vi "CTRE_Phoenix_MotorControl_ConfigAllSettingsEnhanced.vi"(6 "timeoutMs":i32=50, 7 "Force Write":bool, 8 "error in (no error)":errorcluster, 10 "Enhanced Motor Controller Configurables":T1={"Base Configurables"={"openLoopRamp"=0.0, "closedLoopRamp"=0.0, "peakOutputForward"=1.0, "peakOutputReverse"=-1.0, "nominalOutputForward"=0.0, "nominalOutputReverse"=0.0, "neutralDeadband"=0.04, "voltageCompSaturation"=0.0, "voltageMeasurementFilter"=32, "velocityMeasurementPeriod"=100, "velocityMeasurementWindow"=64, "forwardSoftLimitThreshold"=0, "reverseSoftLimitThreshold"=0, "forwardSoftLimitEnable"=FALSE, "reverseSoftLimitEnable"=FALSE, "slot0"={"P"=0.0, "I"=0.0, "D"=0.0, "F"=0.0, "integralZone"=0.0, "allowableClosedLoopError"=0, "maxIntegralAccumulator"=0.0, "closedLoopPeakOutput"=1.0, "closedLoopPeriod"=1}, "slot1"={"P"=0.0, "I"=0.0, "D"=0.0, "F"=0.0, "integralZone"=0.0, "allowableClosedLoopError"=0, "maxIntegralAccumulator"=0.0, "closedLoopPeakOutput"=1.0, "closedLoopPeriod"=1}, "slot2"={"P"=0.0, "I"=0.0, "D"=0.0, "F"=0.0, "integralZone"=0.0, "allowableClosedLoopError"=0, "maxIntegralAccumulator"=0.0, "closedLoopPeakOutput"=1.0, "closedLoopPeriod"=1}, "slot3"={"P"=0.0, "I"=0.0, "D"=0.0, "F"=0.0, "integralZone"=0.0, "allowableClosedLoopError"=0, "maxIntegralAccumulator"=0.0, "closedLoopPeakOutput"=1.0, "closedLoopPeriod"=1}, "auxPIDPolarity"=FALSE, "remoteFilter0"={"remoteSensorDeviceID"=0, "remoteSensorSource"=enum."Off"}, "remoteFilter1"={"remoteSensorDeviceID"=0, "remoteSensorSource"=enum."Off"}, "motionCruiseVelocity"=0, "motionAcceleration"=0, "motionProfileTrajectoryPeriod"=0, "feedbackNotContinuous"=FALSE, "remoteSensorClosedLoopDisableNeutralOnLOS"=FALSE, "clearPositionOnLimitF"=FALSE, "clearPositionOnLimitR"=FALSE, "clearPositionOnQuadIdx"=FALSE, "limitSwitchDisableNeutralOnLOS"=FALSE, "softLimitDisableNeutralOnLOS"=FALSE, "pulseWidthPeriod_EdgesPerRot"=1, "pulseWidthPeriod_FilterWindowSz"=1, "customParam"={"customParam0"=0, "customParam1"=0}}, "primaryPID"={"selectedFeedbackCoefficient"=1.0, "selectedFeedbackSensor"=0}, "auxiliaryPID"={"selectedFeedbackCoefficient"=1.0, "selectedFeedbackSensor"=0}, "sum0Term"=0, "sum1Term"=0, "diff0Term"=0, "diff1Term"=0, "forwardLimitSwitchNormal"=enum."Normally Open", "reverseLimitSwitchNormal"=enum."Normally Open", "forwardLimitSwitchDeviceID"=0, "reverseLimitSwitchDeviceID"=0, "forwardLimitSwitchSource"=enum."Feedback Connector", "reverseLimitSwitchSource"=enum."Feedback Connector", "peakCurrentLimit"=1, "peakCurrentDuration"=1, "continuousCurrentLimit"=1} {"diff1Term" items=["QuadEncoder"=0, "Analog"=2, "Tachometer"=4, "Pulse Width Encoded Position"=8, "Remote Source 0"=11, "Remote Source 1"=12, "Software Emulated"=15]; "diff0Term" items=["QuadEncoder"=0, "Analog"=2, "Tachometer"=4, "Pulse Width Encoded Position"=8, "Remote Source 0"=11, "Remote Source 1"=12, "Software Emulated"=15]; "sum1Term" items=["QuadEncoder"=0, "Analog"=2, "Tachometer"=4, "Pulse Width Encoded Position"=8, "Remote Source 0"=11, "Remote Source 1"=12, "Software Emulated"=15]; "sum0Term" items=["QuadEncoder"=0, "Analog"=2, "Tachometer"=4, "Pulse Width Encoded Position"=8, "Remote Source 0"=11, "Remote Source 1"=12, "Software Emulated"=15]; "auxiliaryPID"."selectedFeedbackSensor" items=["QuadEncoder"=0, "Analog"=2, "Tachometer"=4, "Pulse Width Encoded Position"=8, "Sensor Sum (S0 + S1)"=9, "Sensor Difference (D0 - D1)"=10, "Remote Source 0"=11, "Remote Source 1"=12, "Software Emulated"=15]; "primaryPID"."selectedFeedbackSensor" items=["QuadEncoder"=0, "Analog"=2, "Tachometer"=4, "Pulse Width Encoded Position"=8, "Sensor Sum (S0 + S1)"=9, "Sensor Difference (D0 - D1)"=10, "Remote Source 0"=11, "Remote Source 1"=12, "Software Emulated"=15]; "Base Configurables"."velocityMeasurementPeriod" items=["Period_1ms"=1, "Period_2ms"=2, "Period_5ms"=5, "Period_10ms"=10, "Period_20ms"=20, "Period_25ms"=25, "Period_50ms"=50, "Period_100ms"=100]}, 11 "PhoenixMotorControlDevRef":T12={"DeviceStatus"={"status"=FALSE, "code"=0, "source"=""}, "Type"=enum."PWM", "PWM"={"PWM Channel"=enum."PWM 1", "DeadBand"={"Name"="", "maxPositivePwm"=0, "minPositivePwm"=0, "centerPwm"=0, "maxNegativePwm"=0, "minNegativePwm"=0, "angularRange"=0}}, "CAN"={"Device Number"=0, "SetOutput VI Ref"=variant(enum8{"Percent VBus", "Current", "Speed", "Position", "Voltage"} enum."Percent VBus"), "GetOutput VI Ref"=variant(refnum<k1> refnum), "Enable VI Ref"=variant(dbl 12.0), "Disable VI Ref"=variant(enum8{"Percent VBus", "Speed", "Position", "Slave", "Unchanged / Invalid", "Voltage Compensation", "Current", "Motion Profile"} enum."Percent VBus"), "Data"=variant}, "Invert"=FALSE, "DIO PWM"={"PWM \"Enable\" Channel"=enum."Invalid", "DIOChannel"=enum."Invalid", "PWM Rate"=0.0}}) -> (0 "error out":errorcluster, 3 "PhoenixMotorControlDevRef":T12={"DeviceStatus"={"status"=FALSE, "code"=0, "source"=""}, "Type"=enum."PWM", "PWM"={"PWM Channel"=enum."PWM 1", "DeadBand"={"Name"="", "maxPositivePwm"=0, "minPositivePwm"=0, "centerPwm"=0, "maxNegativePwm"=0, "minNegativePwm"=0, "angularRange"=0}}, "CAN"={"Device Number"=0, "SetOutput VI Ref"=variant(enum8{"Percent VBus", "Current", "Speed", "Position", "Voltage"} enum."Percent VBus"), "GetOutput VI Ref"=variant(refnum<k1> refnum), "Enable VI Ref"=variant(dbl 12.0), "Disable VI Ref"=variant(enum8{"Percent VBus", "Speed", "Position", "Slave", "Unchanged / Invalid", "Voltage Compensation", "Current", "Motion Profile"} enum."Percent VBus"), "Data"=variant}, "Invert"=FALSE, "DIO PWM"={"PWM \"Enable\" Channel"=enum."Invalid", "DIOChannel"=enum."Invalid", "PWM Rate"=0.0}})   [LabVIEW 2017]
doc: "Configures all slot persistant settings\n\n<b> Enhanced Motor Controller Configurables </b> Cluster of all settinsg to be configured"
uses:
  <vilib>/Rock Robotics/WPI/MotorControl/WPI_MotorControlDeviceRef.ctl
  <vilib>/Rock Robotics/WPI/MotorControl/WPI_MotorControlType.ctl
  <vilib>/Rock Robotics/SystemInterfaces/DIO/FPGA_DIOPWMChannel.ctl
  <vilib>/Rock Robotics/WPI/PWM/WPI_PWMDeadband.ctl
  <vilib>/Rock Robotics/SystemInterfaces/DIO/FPGA_DIOChannel.ctl
  <vilib>/Rock Robotics/WPI/ThirdParty/Phoenix-LabVIEW/Motor Controller/Controls/CTRE_Phoenix_MotorControl_EnhancedMotorControllerConfigurables.ctl
  <vilib>/Rock Robotics/WPI/ThirdParty/Phoenix-LabVIEW/Motor Controller/Controls/CTRE_Phoenix_MotorControl_BaseConfigurables.ctl
  <vilib>/Rock Robotics/WPI/ThirdParty/Phoenix-LabVIEW/Motor Controller/Controls/CTRE_Phoenix_MotorControl_VelocityMeasurementPeriod.ctl
  <vilib>/Rock Robotics/WPI/ThirdParty/Phoenix-LabVIEW/Motor Controller/Controls/CTRE_Phoenix_MotorControl_SlotStructure.ctl
  <vilib>/Rock Robotics/WPI/ThirdParty/Phoenix-LabVIEW/Motor Controller/Controls/CTRE_Phoenix_MotorControl_FilterStruct.ctl
  <vilib>/Rock Robotics/WPI/ThirdParty/Phoenix-LabVIEW/Motor Controller/Controls/CTRE_Phoenix_MotorControl_RemoteSourceType.ctl
  <vilib>/Rock Robotics/WPI/ThirdParty/Phoenix-LabVIEW/Controls/CTRE_Phoenix_CustomParamConfiguration.ctl
  <vilib>/Rock Robotics/WPI/ThirdParty/Phoenix-LabVIEW/Motor Controller/Controls/CTRE_Phoenix_MotorControl_FeedbackDevice.ctl
  <vilib>/Rock Robotics/WPI/ThirdParty/Phoenix-LabVIEW/Motor Controller/Controls/CTRE_Phoenix_MotorControl_SensorTermFeedbackDevice_Enhanced.ctl
  <vilib>/Rock Robotics/WPI/ThirdParty/Phoenix-LabVIEW/Motor Controller/Controls/CTRE_Phoenix_MotorControl_LimitSwitchNormal.ctl
  <vilib>/Rock Robotics/WPI/ThirdParty/Phoenix-LabVIEW/Motor Controller/Controls/CTRE_Phoenix_MotorControl_LimitSwitchSource_Local.ctl
panel:
  # "Sum and Diff terms are ways to select more than one sensor as a feedback device. \n Sum 0 is the first feedback device to be used for the Sum term.\n Sum 1 is the feedback device to be added to Sum 0 for the Sum term.\n Diff 0 and Diff 1 work in a similar manner."
  # "These are only applicable\nif using a remote limit switch.\n\nLocal limit switches/no limit\nswitches do not use this."
  # "Current is below Continuous threshold AND\n\n(Requested output is weaker** than applied motor\noutput OR is in the opposite direction).\n/\nMotor output is set to requested output."
  # "Current is above Peak* Threshold for Peak Duration.\n/\nReduce motor output (towards neutral)."
  # "Current is below Continuous threshold.\n/\nRamp motor output towards requested output."
  # "Current is above Continuous threshold.\n/\nReduce motor output (towards neutral)."
  # "Current Limiting is NOT enabled\nby default.\nCall this VI to enable."
  # "*If the configured Peak Threshold is less than the Continuous Threshold, the applied Peak Threshold is set equal to the Configured Continuous Threshold in firmware.\n** Both requested output and applied motor output are in the same direction, and requested output is closer to neutral."
  # "False: Primary Output = PID[0] + PID[1]  ---  Auxiliary Output = PID[0] - PID[1]\nTrue:  Primary Output = PID[0] - PID[1] --- Auxiliary Output = PID[0] + PID[1]"
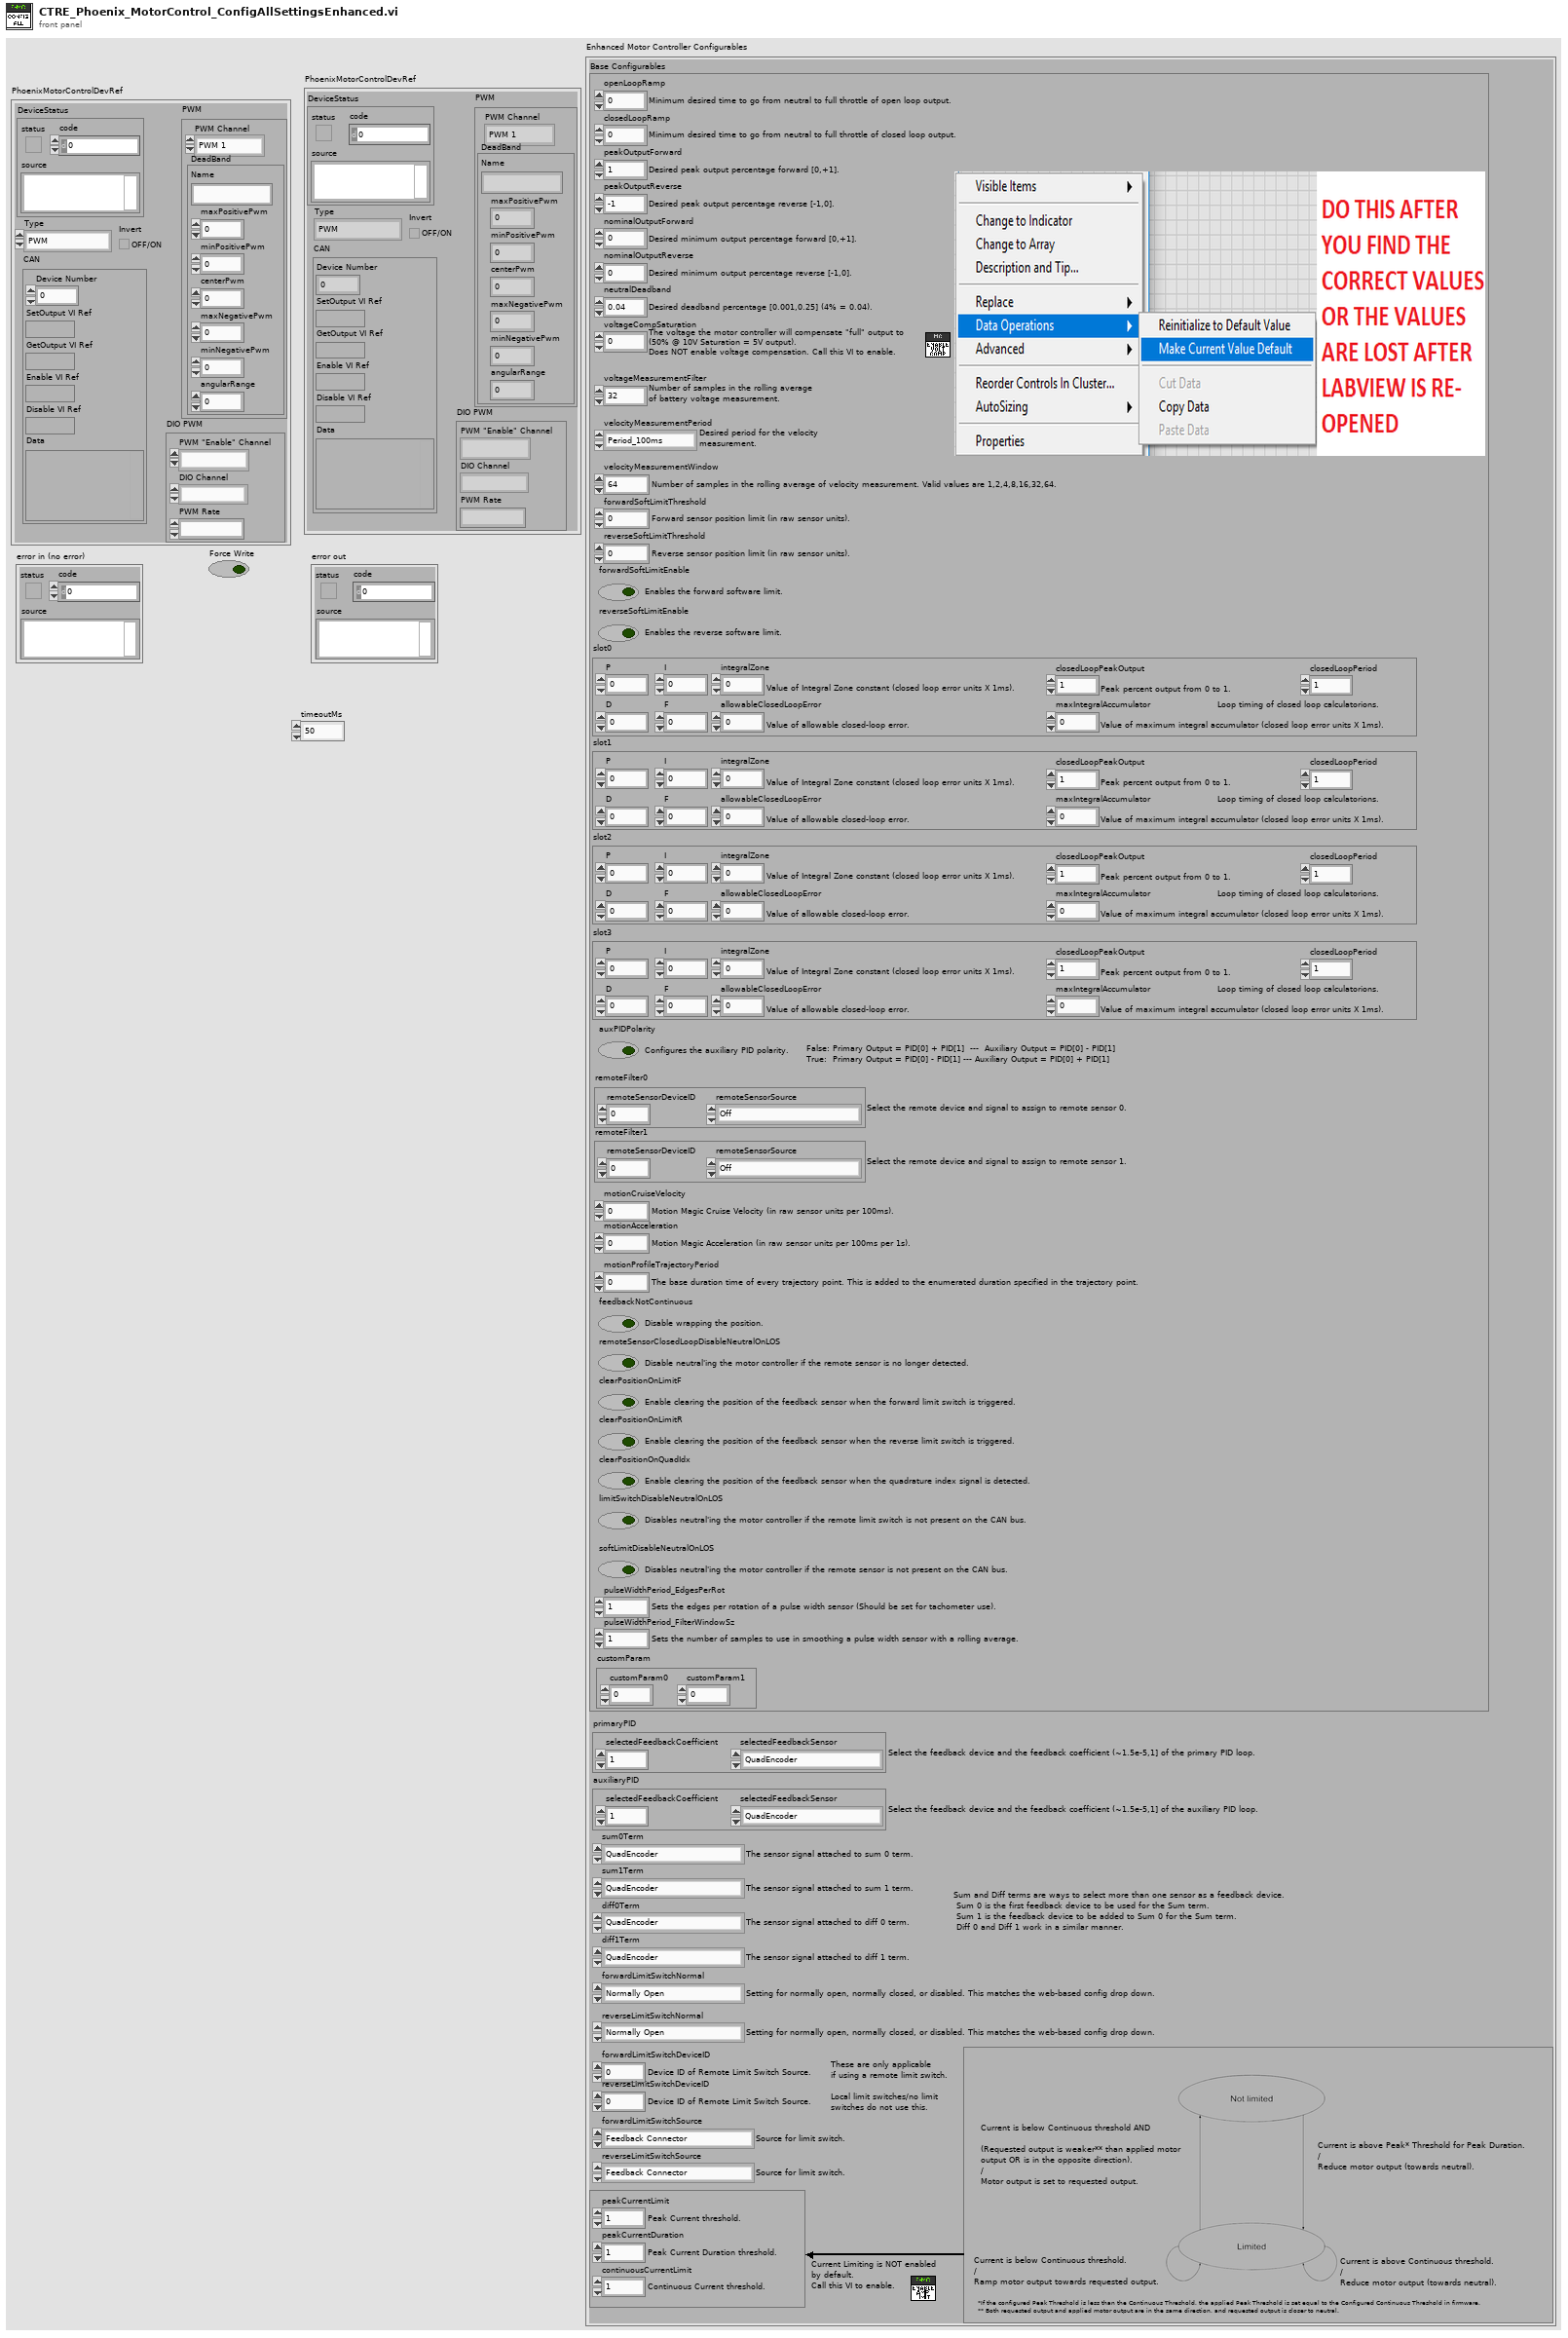
[diagram p1: front panel]
types:
  T1 = typedef "CTRE_Phoenix_MotorControl_EnhancedMotorControllerConfigurables.ctl" = cluster{"Base Configurables":T2, "primaryPID":cluster{"selectedFeedbackCoefficient":dbl, "selectedFeedbackSensor":T8}, "auxiliaryPID":cluster{"selectedFeedbackCoefficient":dbl, "selectedFeedbackSensor":T8}, "sum0Term":T9, "sum1Term":T9, "diff0Term":T9, "diff1Term":T9, "forwardLimitSwitchNormal":T10, "reverseLimitSwitchNormal":T10, "forwardLimitSwitchDeviceID":i32, "reverseLimitSwitchDeviceID":i32, "forwardLimitSwitchSource":T11, "reverseLimitSwitchSource":T11, "peakCurrentLimit":i32, "peakCurrentDuration":i32, "continuousCurrentLimit":i32}
  T2 = typedef "CTRE_Phoenix_MotorControl_BaseConfigurables.ctl" = cluster{"openLoopRamp":dbl, "closedLoopRamp":dbl, "peakOutputForward":dbl, "peakOutputReverse":dbl, "nominalOutputForward":dbl, "nominalOutputReverse":dbl, "neutralDeadband":dbl, "voltageCompSaturation":dbl, "voltageMeasurementFilter":i32, "velocityMeasurementPeriod":T3, "velocityMeasurementWindow":i32, "forwardSoftLimitThreshold":i32, "reverseSoftLimitThreshold":i32, "forwardSoftLimitEnable":bool, "reverseSoftLimitEnable":bool, "slot0":T4, "slot1":T4, "slot2":T4, "slot3":T4, "auxPIDPolarity":bool, "remoteFilter0":T5, "remoteFilter1":T5, "motionCruiseVelocity":i32, "motionAcceleration":i32, "motionProfileTrajectoryPeriod":i32, "feedbackNotContinuous":bool, "remoteSensorClosedLoopDisableNeutralOnLOS":bool, "clearPositionOnLimitF":bool, "clearPositionOnLimitR":bool, "clearPositionOnQuadIdx":bool, "limitSwitchDisableNeutralOnLOS":bool, "softLimitDisableNeutralOnLOS":bool, "pulseWidthPeriod_EdgesPerRot":i32, "pulseWidthPeriod_FilterWindowSz":i32, "customParam":T7}
  T3 = typedef "CTRE_Phoenix_MotorControl_VelocityMeasurementPeriod.ctl" = u16
  T4 = typedef "CTRE_Phoenix_MotorControl_SlotStructure.ctl" = cluster{"P":dbl, "I":dbl, "D":dbl, "F":dbl, "integralZone":dbl, "allowableClosedLoopError":i32, "maxIntegralAccumulator":dbl, "closedLoopPeakOutput":dbl, "closedLoopPeriod":i32}
  T5 = typedef "CTRE_Phoenix_MotorControl_FilterStruct.ctl" = cluster{"remoteSensorDeviceID":u8, "remoteSensorSource":T6}
  T6 = typedef "CTRE_Phoenix_MotorControl_RemoteSourceType.ctl" = enum16{"Off", "Talon SRX Selected Sensor", "Pigeon IMU Yaw", "Pigeon IMU Pitch", "Pigeon IMU Roll", "CANifier Quadrature", "CANifier PWM Input 0", "CANifier PWM Input 1", "CANifier PWM Input 2", "CANifier PWM Input 3", "Gadgeteer Pigeon Yaw", "Gadgeteer Pigeon Pitch", "Gadgeteer Pigeon Roll"}
  T7 = typedef "CTRE_Phoenix_CustomParamConfiguration.ctl" = cluster{"customParam0":i32, "customParam1":i32}
  T8 = typedef "CTRE_Phoenix_MotorControl_FeedbackDevice.ctl" = i8
  T9 = typedef "CTRE_Phoenix_MotorControl_SensorTermFeedbackDevice_Enhanced.ctl" = i8
  T10 = typedef "CTRE_Phoenix_MotorControl_LimitSwitchNormal.ctl" = enum16{"Normally Open", "Normally Closed", "Disabled"}
  T11 = typedef "CTRE_Phoenix_MotorControl_LimitSwitchSource_Local.ctl" = enum16{"Feedback Connector", "Remote Talon SRX", "Remote CANifier", "Deactivated"}
  T12 = typedef "WPI_MotorControlDeviceRef.ctl" = cluster{"DeviceStatus":errorcluster, "Type":T13, "PWM":cluster{"PWM Channel":T14, "DeadBand":T15}, "CAN":cluster{"Device Number":u8, "SetOutput VI Ref":variant, "GetOutput VI Ref":variant, "Enable VI Ref":variant, "Disable VI Ref":variant, "Data":variant}, "Invert":bool, "DIO PWM":cluster{"PWM \"Enable\" Channel":T14, "DIOChannel":T16, "PWM Rate":dbl}}
  T13 = typedef "WPI_MotorControlType.ctl" = enum16{"PWM", "CAN", "DIO PWM"}
  T14 = typedef "FPGA_DIOPWMChannel.ctl" = enum8{"PWM 0", "PWM 1", "PWM 2", "PWM 3", "PWM 4", "PWM 5", "PWM 6", "PWM 7", "PWM 8", "PWM 9", "PWM MXP 0", "PWM MXP 1", "PWM MXP 2", "PWM MXP 3", "PWM MXP 4", "PWM MXP 5", "PWM MXP 6", "PWM MXP 7", "PWM MXP 8", "PWM MXP 9", "Invalid"}
  T15 = typedef "WPI_PWMDeadband.ctl" = cluster{"Name":string, "maxPositivePwm":i32, "minPositivePwm":i32, "centerPwm":i32, "maxNegativePwm":i32, "minNegativePwm":i32, "angularRange":u16}
  T16 = typedef "FPGA_DIOChannel.ctl" = enum8{"DIO 0", "DIO 1", "DIO 2", "DIO 3", "DIO 4", "DIO 5", "DIO 6", "DIO 7", "DIO 8", "DIO 9", "DIO MXP 0", "DIO MXP 1", "DIO MXP 2", "DIO MXP 3", "DIO MXP 4", "DIO MXP 5", "DIO MXP 6", "DIO MXP 7", "DIO MXP 8", "DIO MXP 9", "DIO MXP 10", "DIO MXP 11", "DIO MXP 12", "DIO MXP 13", "DIO MXP 14", "DIO MXP 15", "SPI Port CS1", "SPI Port CS2", "SPI Port CS3", "SPI Port MISO", "SPI Port MOSI", "Invalid"}
  T17 = cluster{"Base Configurables":cluster{"openLoopRamp":bool, "closedLoopRamp":bool, "peakOutputForward":bool, "peakOutputReverse":bool, "nominalOutputForward":bool, "nominalOutputReverse":bool, "neutralDeadband":bool, "voltageCompSaturation":bool, "voltageMeasurementFilter":bool, "velocityMeasurementPeriod":bool, "velocityMeasurementWindow":bool, "forwardSoftLimitThreshold":bool, "reverseSoftLimitThreshold":bool, "forwardSoftLimitEnable":bool, "reverseSoftLimitEnable":bool, "slot0":cluster{"P":bool, "I":bool, "D":bool, "F":bool, "integralZone":bool, "allowableClosedLoopError":bool, "maxIntegralAccumulator":bool, "closedLoopPeakOutput":bool, "closedLoopPeriod":bool}, "slot1":cluster{"P":bool, "I":bool, "D":bool, "F":bool, "integralZone":bool, "allowableClosedLoopError":bool, "maxIntegralAccumulator":bool, "closedLoopPeakOutput":bool, "closedLoopPeriod":bool}, "slot2":cluster{"P":bool, "I":bool, "D":bool, "F":bool, "integralZone":bool, "allowableClosedLoopError":bool, "maxIntegralAccumulator":bool, "closedLoopPeakOutput":bool, "closedLoopPeriod":bool}, "slot3":cluster{"P":bool, "I":bool, "D":bool, "F":bool, "integralZone":bool, "allowableClosedLoopError":bool, "maxIntegralAccumulator":bool, "closedLoopPeakOutput":bool, "closedLoopPeriod":bool}, "auxPIDPolarity":bool, "remoteFilter0":cluster{"remoteSensorDeviceID":bool, "remoteSensorSource":bool}, "remoteFilter1":cluster{"remoteSensorDeviceID":bool, "remoteSensorSource":bool}, "motionCruiseVelocity":bool, "motionAcceleration":bool, "motionProfileTrajectoryPeriod":bool, "feedbackNotContinuous":bool, "remoteSensorClosedLoopDisableNeutralOnLOS":bool, "clearPositionOnLimitF":bool, "clearPositionOnLimitR":bool, "clearPositionOnQuadIdx":bool, "limitSwitchDisableNeutralOnLOS":bool, "softLimitDisableNeutralOnLOS":bool, "pulseWidthPeriod_EdgesPerRot":bool, "pulseWidthPeriod_FilterWindowSz":bool, "customParam":cluster{"customParam0":bool, "customParam1":bool}}, "primaryPID":cluster{"selectedFeedbackCoefficient":bool, "selectedFeedbackSensor":bool}, "auxiliaryPID":cluster{"selectedFeedbackCoefficient":bool, "selectedFeedbackSensor":bool}, "sum0Term":bool, "sum1Term":bool, "diff0Term":bool, "diff1Term":bool, "forwardLimitSwitchNormal":bool, "reverseLimitSwitchNormal":bool, "forwardLimitSwitchDeviceID":bool, "reverseLimitSwitchDeviceID":bool, "forwardLimitSwitchSource":bool, "reverseLimitSwitchSource":bool, "peakCurrentLimit":bool, "peakCurrentDuration":bool, "continuousCurrentLimit":bool}
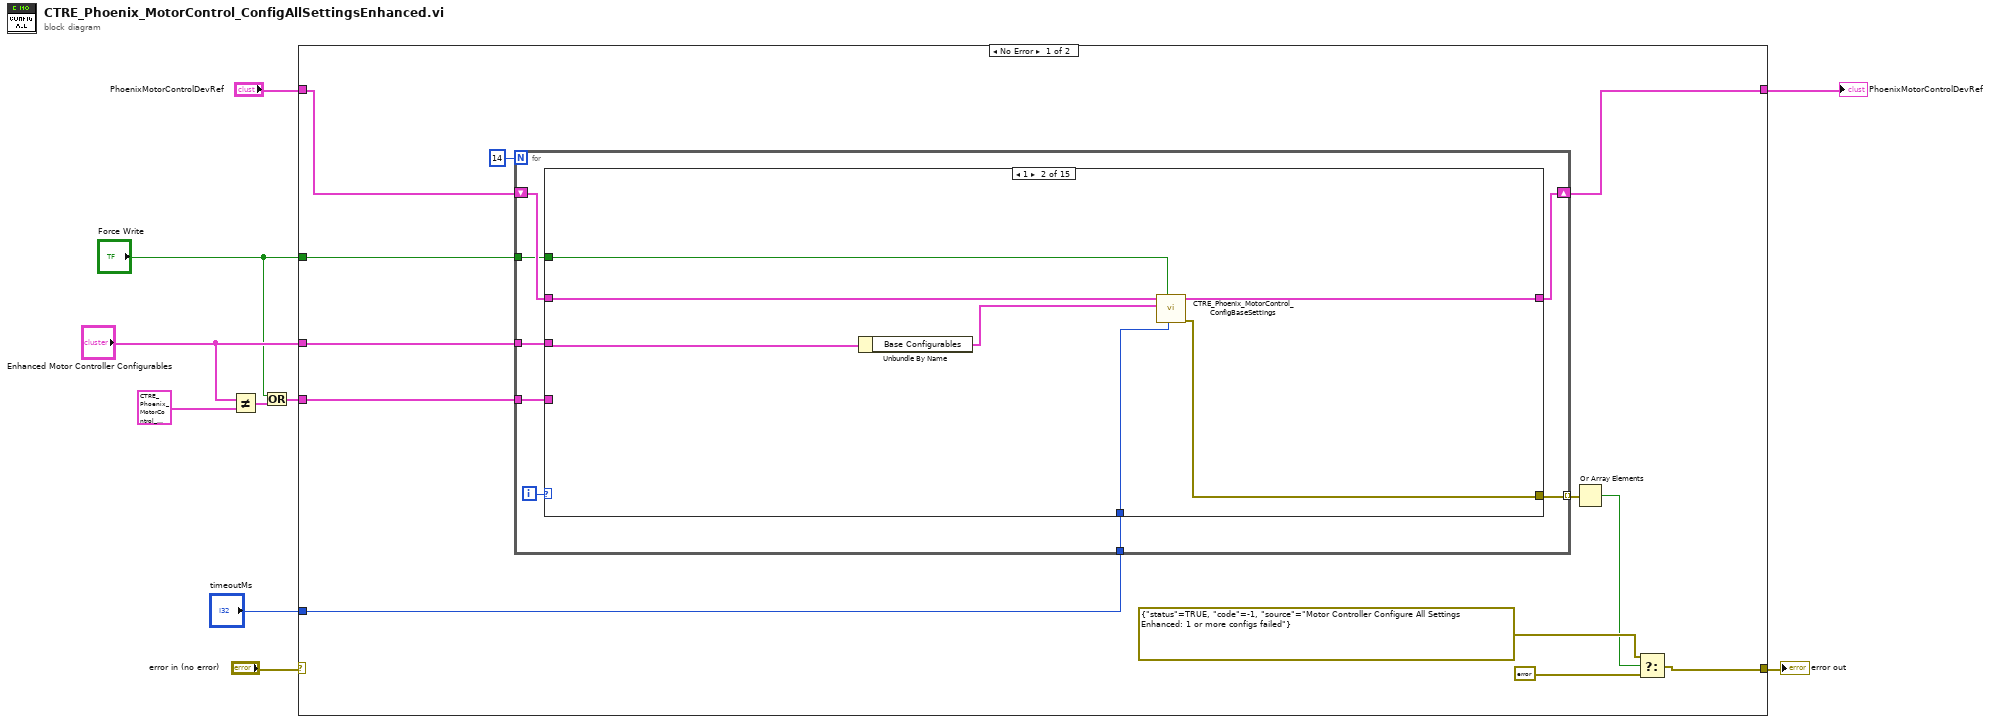
[diagram p0: block diagram]
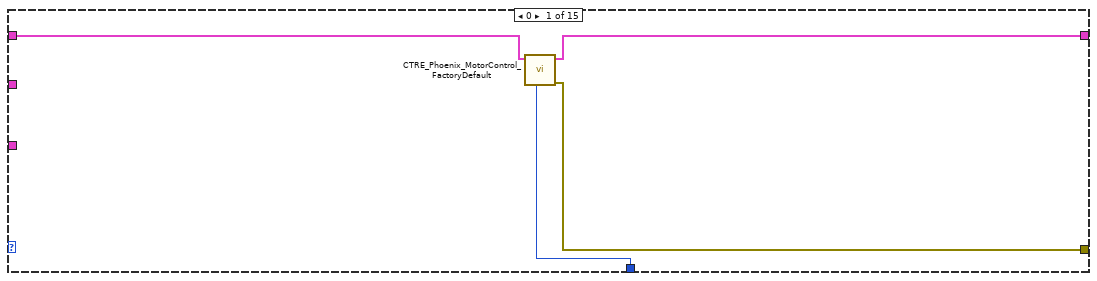
[diagram p2: hidden frame]
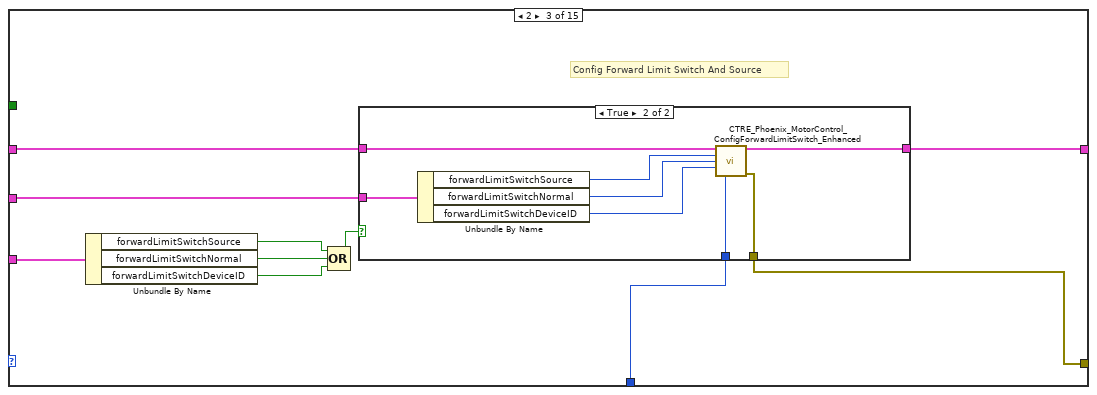
[diagram p3: hidden frame]
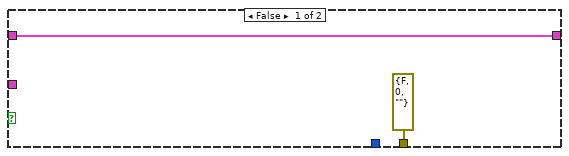
[diagram p4: hidden frame]
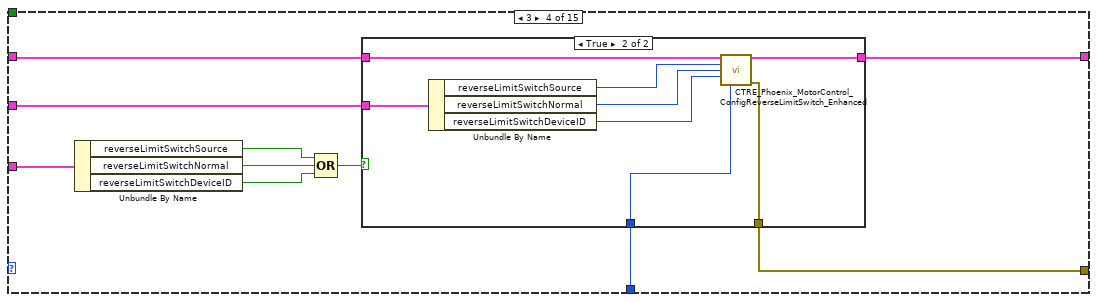
[diagram p5: hidden frame]
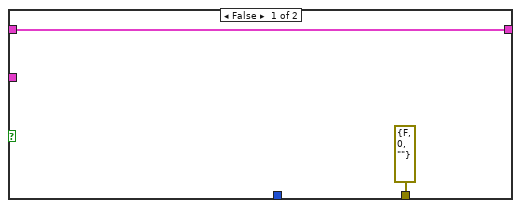
[diagram p6: hidden frame]
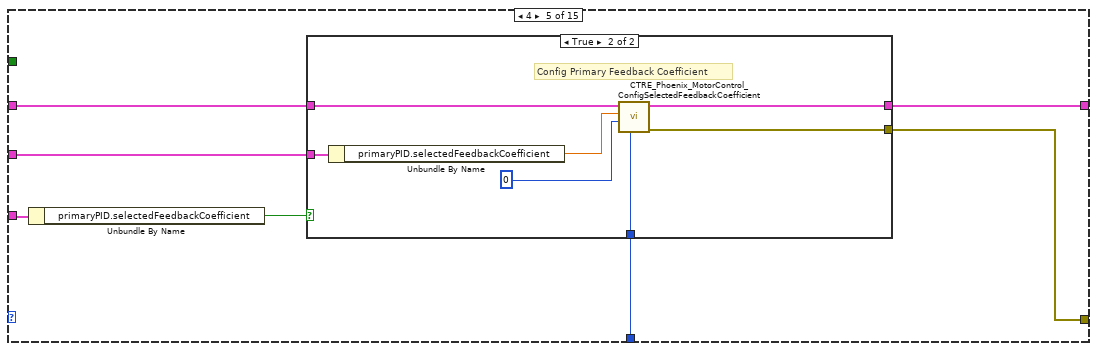
[diagram p7: hidden frame]
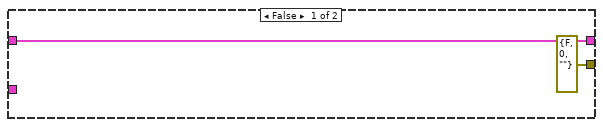
[diagram p8: hidden frame]
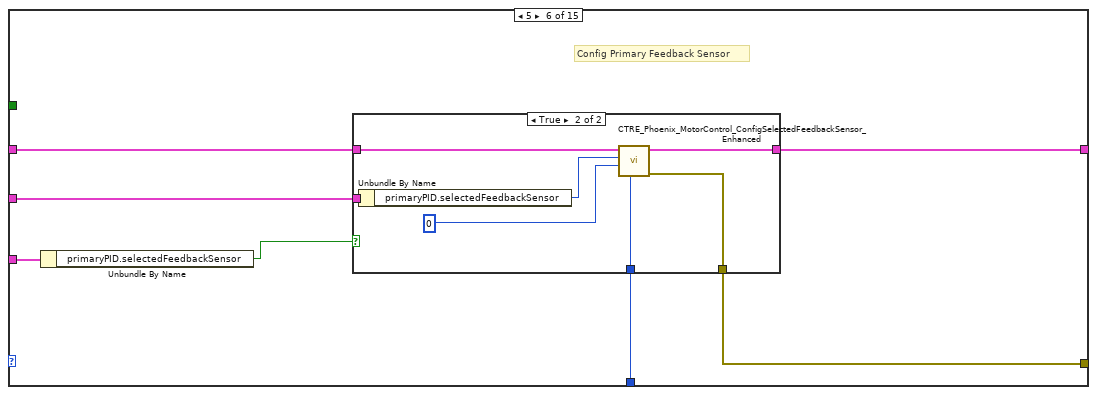
[diagram p9: hidden frame]
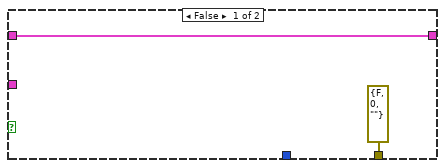
[diagram p10: hidden frame]
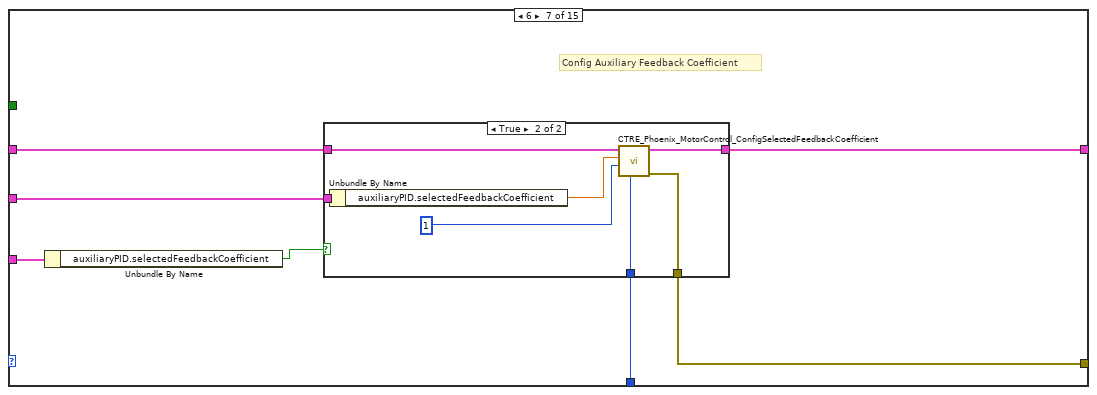
[diagram p11: hidden frame]
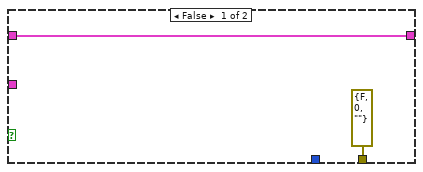
[diagram p12: hidden frame]
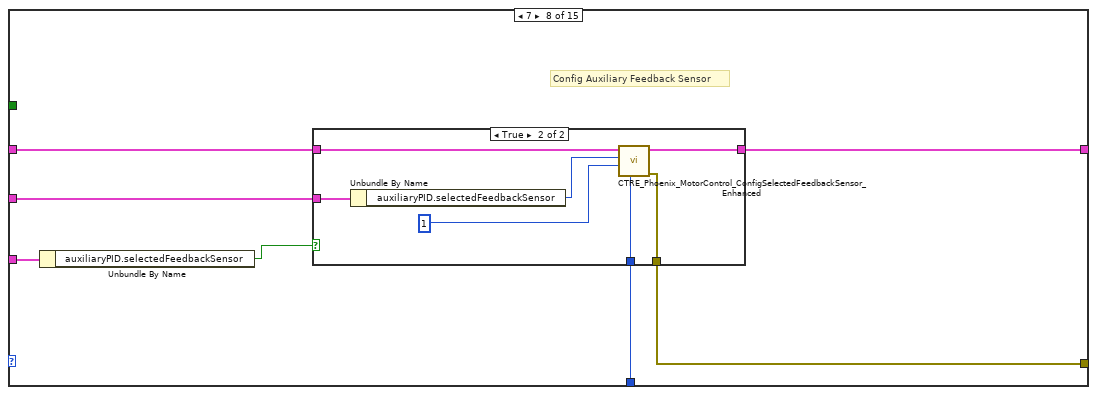
[diagram p13: hidden frame]
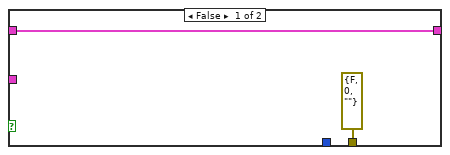
[diagram p14: hidden frame]
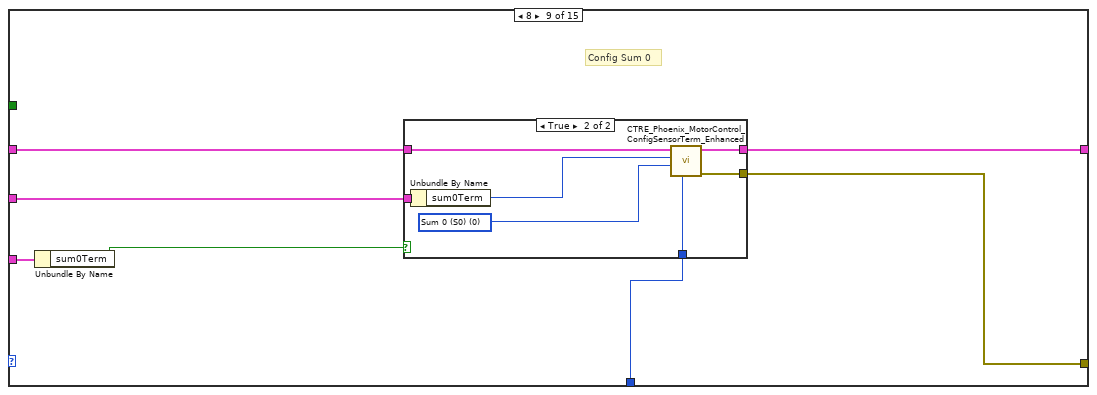
[diagram p15: hidden frame]
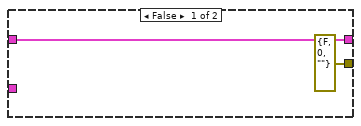
[diagram p16: hidden frame]
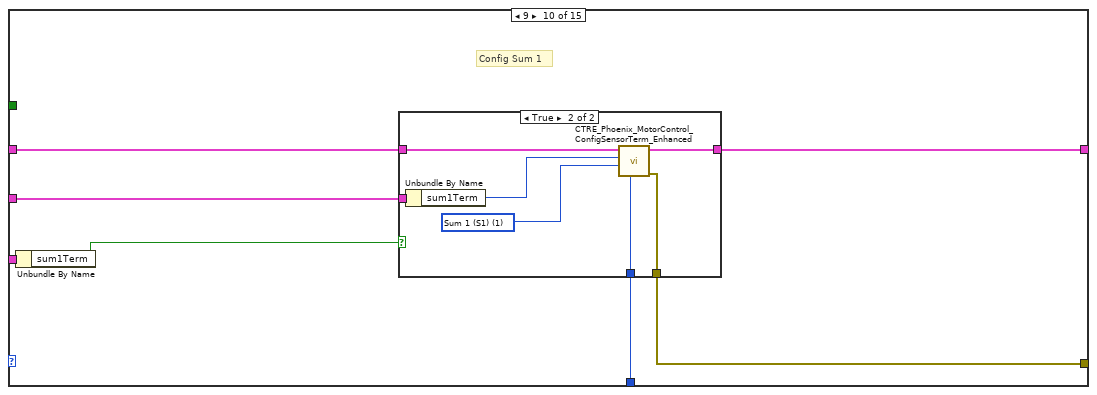
[diagram p17: hidden frame]
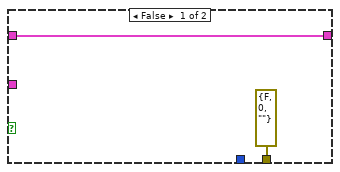
[diagram p18: hidden frame]
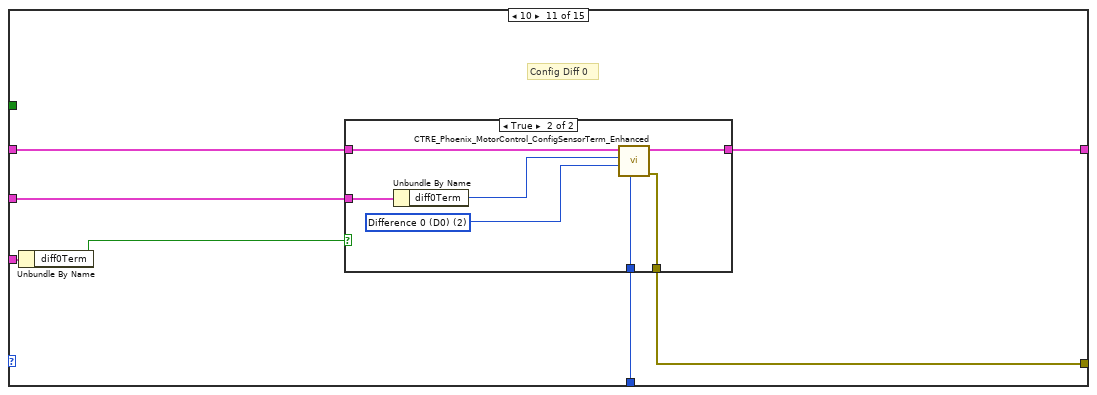
[diagram p19: hidden frame]
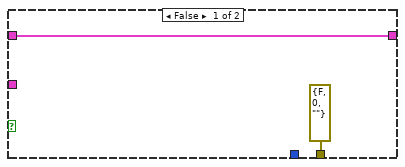
[diagram p20: hidden frame]
diagram:
  n1 = Not Equal?(x="Enhanced Motor Controller Configurables", y=T1 {"Base Configurables"={"openLoopRamp"=0.0, "closedLoopRamp"=0.0, "peakOutputForward"=1.0, "peakOutputReverse"=-1.0, "nominalOutputForward"=0.0, "nominalOutputReverse"=0.0, "neutralDeadband"=0.04, "voltageCompSaturation"=0.0, "voltageMeasurementFilter"=32, "velocityMeasurementPeriod"=100, "velocityMeasurementWindow"=64, "forwardSoftLimitThreshold"=0, "reverseSoftLimitThreshold"=0, "forwardSoftLimitEnable"=FALSE, "reverseSoftLimitEnable"=FALSE, "slot0"={"P"=0.0, "I"=0.0, "D"=0.0, "F"=0.0, "integralZone"=0.0, "allowableClosedLoopError"=0, "maxIntegralAccumulator"=0.0, "closedLoopPeakOutput"=1.0, "closedLoopPeriod"=1}, "slot1"={"P"=0.0, "I"=0.0, "D"=0.0, "F"=0.0, "integralZone"=0.0, "allowableClosedLoopError"=0, "maxIntegralAccumulator"=0.0, "closedLoopPeakOutput"=1.0, "closedLoopPeriod"=1}, "slot2"={"P"=0.0, "I"=0.0, "D"=0.0, "F"=0.0, "integralZone"=0.0, "allowableClosedLoopError"=0, "maxIntegralAccumulator"=0.0, "closedLoopPeakOutput"=1.0, "closedLoopPeriod"=1}, "slot3"={"P"=0.0, "I"=0.0, "D"=0.0, "F"=0.0, "integralZone"=0.0, "allowableClosedLoopError"=0, "maxIntegralAccumulator"=0.0, "closedLoopPeakOutput"=1.0, "closedLoopPeriod"=1}, "auxPIDPolarity"=FALSE, "remoteFilter0"={"remoteSensorDeviceID"=0, "remoteSensorSource"=enum."Off"}, "remoteFilter1"={"remoteSensorDeviceID"=0, "remoteSensorSource"=enum."Off"}, "motionCruiseVelocity"=0, "motionAcceleration"=0, "motionProfileTrajectoryPeriod"=0, "feedbackNotContinuous"=FALSE, "remoteSensorClosedLoopDisableNeutralOnLOS"=FALSE, "clearPositionOnLimitF"=FALSE, "clearPositionOnLimitR"=FALSE, "clearPositionOnQuadIdx"=FALSE, "limitSwitchDisableNeutralOnLOS"=FALSE, "softLimitDisableNeutralOnLOS"=FALSE, "pulseWidthPeriod_EdgesPerRot"=1, "pulseWidthPeriod_FilterWindowSz"=1, "customParam"={"customParam0"=0, "customParam1"=0}}, "primaryPID"={"selectedFeedbackCoefficient"=1.0, "selectedFeedbackSensor"=0}, "auxiliaryPID"={"selectedFeedbackCoefficient"=1.0, "selectedFeedbackSensor"=0}, "sum0Term"=0, "sum1Term"=0, "diff0Term"=0, "diff1Term"=0, "forwardLimitSwitchNormal"=enum."Normally Open", "reverseLimitSwitchNormal"=enum."Normally Open", "forwardLimitSwitchDeviceID"=0, "reverseLimitSwitchDeviceID"=0, "forwardLimitSwitchSource"=enum."Feedback Connector", "reverseLimitSwitchSource"=enum."Feedback Connector", "peakCurrentLimit"=1, "peakCurrentDuration"=1, "continuousCurrentLimit"=1}) -> (x != y?=w2:T17)
  n2 = Or(x="Force Write", y=w2) -> (x .or. y?=w3:T17)
  n3 = case shown="No Error" "error in (no error)" {
    selector: "error in (no error)" -> [_ w246]
    tunnel: [w22 w246] -> w10
    tunnel: "PhoenixMotorControlDevRef" -> [w18 w245]
    tunnel: [w13 w245] -> w6
    tunnel: "timeoutMs" -> [w17 _]
    tunnel: "Enhanced Motor Controller Configurables" -> [w19 _]
    tunnel: "Force Write" -> [w12 _]
    tunnel: w3 -> [w11 _]
    frame No Error {
      n4 = for {
        N: 14 -> [_]
        tunnel: w19 -> [w30]
        tunnel: w17 -> [w28]
        tunnel: [w26] -> w16 mode=indexing
        shift-right: [w27] -> w13
        shift-left: w18 -> [w29]
        tunnel: w12 -> [w24]
        tunnel: w11 -> [w23]
        i -> [w25]
        n5 = case shown="1" w25 {
          tunnel: w29 -> [w34 w40 w50 w71 w87 w103 w120 w135 w151 w167 w184 w200 w218 w233 w244]
          tunnel: [w33 w41 w47 w67 w86 w102 w119 w136 w150 w165 w183 w197 w217 w232 w244] -> w27
          tunnel: w28 -> [w32 w37 w49 w69 w84 w101 w117 w132 w149 w166 w182 w198 w215 w230 _]
          tunnel: w30 -> [_ w39 w51 w70 w88 w104 w118 w134 w152 w168 w180 w199 w216 w234 _]
          tunnel: [w31 w35 w48 w68 w85 w100 w116 w133 w148 w164 w181 w196 w214 w231 errorcluster {"status"=FALSE, "code"=0, "source"=""} ("error out")] -> w26
          tunnel: w24 -> [_ w36 _ _ _ _ _ _ _ _ _ _ _ _ _]
          tunnel: w23 -> [_ _ w46 w66 w83 w99 w115 w131 w147 w163 w179 w195 w213 w229 _]
          frame 0 {
            n6 = call <vilib>:"CTRE_Phoenix_MotorControl_FactoryDefault.vi"("timeoutMs"=w32, "PhoenixMotorControlDevRef"=w34) -> ("error out"=w31:errorcluster, "PhoenixMotorControlDevRef"=w33:T12)  [unwired: 8 in]
          }
          frame 1 {
            n7 = Unbundle By Name(w39) -> ("Base Configurables"=w38:T2)
            n8 = call <vilib>:"CTRE_Phoenix_MotorControl_ConfigBaseSettings.vi"("timeoutMs"=w37, "Force Write"=w36, "Base Configurables"=w38, "PhoenixMotorControlDevRef in"=w40) -> ("error out"=w35:errorcluster, "PhoenixMotorControlDevRef out"=w41:T12)  [unwired: 6 in]
          }
          frame 2 {
            # "Config Forward Limit Switch And Source"
            n9 = Unbundle By Name(w46) -> ("forwardLimitSwitchSource"=w44:bool, "forwardLimitSwitchNormal"=w45:bool, "forwardLimitSwitchDeviceID"=w43:bool)
            n10 = Compound Arithmetic op=OR(w44, w45, w43) -> (w42:bool)
            n11 = case shown="True" w42 {
              tunnel: w51 -> [_ w58]
              tunnel: w50 -> [w53 w57]
              tunnel: w49 -> [_ w56]
              tunnel: [errorcluster {"status"=FALSE, "code"=0, "source"=""} ("error out") w55] -> w48
              tunnel: [w53 w54] -> w47
              frame False {
              }
              frame True {
                n12 = Unbundle By Name(w58) -> ("forwardLimitSwitchSource"=w61:T11, "forwardLimitSwitchNormal"=w60:T10, "forwardLimitSwitchDeviceID"=w59:i32)
                n13 = call <vilib>:"CTRE_Phoenix_MotorControl_ConfigForwardLimitSwitch_Enhanced.vi"("PhoenixMotorControlDevRef"=w57, "Limit Switch Source"=w61, "NormallyOpenOrClosed"=w60, "deviceID"=w59, "timeoutMs"=w56) -> ("PhoenixMotorControlDevRef"=w54:T12, "error out"=w55:errorcluster)  [unwired: 9 in]
              }
            }
          }
          frame 3 {
            n14 = Unbundle By Name(w66) -> ("reverseLimitSwitchSource"=w65:bool, "reverseLimitSwitchNormal"=w64:bool, "reverseLimitSwitchDeviceID"=w63:bool)
            n15 = Compound Arithmetic op=OR(w65, w64, w63) -> (w62:bool)
            n16 = case shown="True" w62 {
              tunnel: w71 -> [w73 w78]
              tunnel: w70 -> [_ w77]
              tunnel: w69 -> [_ w76]
              tunnel: [errorcluster {"status"=FALSE, "code"=0, "source"=""} ("error out") w75] -> w68
              tunnel: [w73 w74] -> w67
              frame False {
              }
              frame True {
                n17 = Unbundle By Name(w77) -> ("reverseLimitSwitchSource"=w81:T11, "reverseLimitSwitchNormal"=w80:T10, "reverseLimitSwitchDeviceID"=w79:i32)
                n18 = call <vilib>:"CTRE_Phoenix_MotorControl_ConfigReverseLimitSwitch_Enhanced.vi"("PhoenixMotorControlDevRef"=w78, "Limit Switch Source"=w81, "NormallyOpenOrClosed"=w80, "deviceID"=w79, "timeoutMs"=w76) -> ("PhoenixMotorControlDevRef"=w74:T12, "error out"=w75:errorcluster)  [unwired: 9 in]
              }
            }
          }
          frame 4 {
            n19 = Unbundle By Name(w83) -> ("primaryPID.selectedFeedbackCoefficient"=w82:bool)
            n20 = case shown="True" w82 {
              tunnel: w88 -> [_ w97]
              tunnel: w87 -> [w90 w96]
              tunnel: [w90 w94] -> w86
              tunnel: [errorcluster {"status"=FALSE, "code"=0, "source"=""} ("error out") w93] -> w85
              tunnel: w84 -> [_ w92]
              frame False {
              }
              frame True {
                # "Config Primary Feedback Coefficient"
                n21 = Unbundle By Name(w97) -> ("primaryPID.selectedFeedbackCoefficient"=w95:dbl)
                n22 = call <vilib>:"CTRE_Phoenix_MotorControl_ConfigSelectedFeedbackCoefficient.vi"("timoutMs"=w92, "pidIdx"=0, "coefficient"=w95, "PhoenixMotorControlDevRef"=w96) -> ("error out"=w93:errorcluster, "PhoenixMotorControlDevRef"=w94:T12)  [unwired: 6 in]
              }
            }
          }
          frame 5 {
            # "Config Primary Feedback Sensor"
            n23 = Unbundle By Name(w99) -> ("primaryPID.selectedFeedbackSensor"=w98:bool)
            n24 = case shown="True" w98 {
              tunnel: w104 -> [_ w113]
              tunnel: w103 -> [w106 w112]
              tunnel: [w106 w111] -> w102
              tunnel: w101 -> [_ w109]
              tunnel: [errorcluster {"status"=FALSE, "code"=0, "source"=""} ("error out") w108] -> w100
              frame False {
              }
              frame True {
                n25 = Unbundle By Name(w113) -> ("primaryPID.selectedFeedbackSensor"=w110:T8)
                n26 = call <vilib>:"CTRE_Phoenix_MotorControl_ConfigSelectedFeedbackSensor_Enhanced.vi"("timeoutMs"=w109, "pidLoopIdx"=0, "Feedback Device"=w110, "PhoenixMotorControlDevRef"=w112) -> ("error out"=w108:errorcluster, "PhoenixMotorControlDevRef"=w111:T12)  [unwired: 6 in]
              }
            }
          }
          frame 6 {
            # "Config Auxiliary Feedback Coefficient"
            n27 = Unbundle By Name(w115) -> ("auxiliaryPID.selectedFeedbackCoefficient"=w114:bool)
            n28 = case shown="True" w114 {
              tunnel: w120 -> [w122 w127]
              tunnel: [w122 w126] -> w119
              tunnel: w118 -> [_ w125]
              tunnel: w117 -> [_ w124]
              tunnel: [errorcluster {"status"=FALSE, "code"=0, "source"=""} ("error out") w123] -> w116
              frame False {
              }
              frame True {
                n29 = Unbundle By Name(w125) -> ("auxiliaryPID.selectedFeedbackCoefficient"=w129:dbl)
                n30 = call <vilib>:"CTRE_Phoenix_MotorControl_ConfigSelectedFeedbackCoefficient.vi"("timoutMs"=w124, "pidIdx"=1, "coefficient"=w129, "PhoenixMotorControlDevRef"=w127) -> ("error out"=w123:errorcluster, "PhoenixMotorControlDevRef"=w126:T12)  [unwired: 6 in]
              }
            }
          }
          frame 7 {
            # "Config Auxiliary Feedback Sensor"
            n31 = Unbundle By Name(w131) -> ("auxiliaryPID.selectedFeedbackSensor"=w130:bool)
            n32 = case shown="True" w130 {
              tunnel: [w138 w143] -> w136
              tunnel: w135 -> [w138 w142]
              tunnel: w134 -> [_ w141]
              tunnel: [errorcluster {"status"=FALSE, "code"=0, "source"=""} ("error out") w140] -> w133
              tunnel: w132 -> [_ w139]
              frame False {
              }
              frame True {
                n33 = Unbundle By Name(w141) -> ("auxiliaryPID.selectedFeedbackSensor"=w145:T8)
                n34 = call <vilib>:"CTRE_Phoenix_MotorControl_ConfigSelectedFeedbackSensor_Enhanced.vi"("timeoutMs"=w139, "pidLoopIdx"=1, "Feedback Device"=w145, "PhoenixMotorControlDevRef"=w142) -> ("error out"=w140:errorcluster, "PhoenixMotorControlDevRef"=w143:T12)  [unwired: 6 in]
              }
            }
          }
          frame 8 {
            # "Config Sum 0"
            n35 = Unbundle By Name(w147) -> ("sum0Term"=w146:bool)
            n36 = case shown="True" w146 {
              tunnel: w152 -> [_ w161]
              tunnel: w151 -> [w154 w160]
              tunnel: [w154 w159] -> w150
              tunnel: w149 -> [_ w156]
              tunnel: [errorcluster {"status"=FALSE, "code"=0, "source"=""} ("error out") w155] -> w148
              frame False {
              }
              frame True {
                w158 = u16 0 items=["Sum 0 (S0)", "Sum 1 (S1)", "Difference 0 (D0)", "Difference 1 (D1)"] ("Sensor Term")
                n37 = Unbundle By Name(w161) -> ("sum0Term"=w157:T9)
                n38 = call <vilib>:"CTRE_Phoenix_MotorControl_ConfigSensorTerm_Enhanced.vi"("timeoutMs"=w156, "Sensor Term"=w158, "Feedback Device"=w157, "PhoenixMotorControlDevRef"=w160) -> ("error out"=w155:errorcluster, "PhoenixMotorControlDevRef"=w159:T12)  [unwired: 6 in]
              }
            }
          }
          frame 9 {
            # "Config Sum 1"
            n39 = Unbundle By Name(w163) -> ("sum1Term"=w162:bool)
            n40 = case shown="True" w162 {
              tunnel: w168 -> [_ w177]
              tunnel: w167 -> [w170 w176]
              tunnel: w166 -> [_ w173]
              tunnel: [w170 w172] -> w165
              tunnel: [errorcluster {"status"=FALSE, "code"=0, "source"=""} ("error out") w171] -> w164
              frame False {
              }
              frame True {
                w174 = u16 1 items=["Sum 0 (S0)", "Sum 1 (S1)", "Difference 0 (D0)", "Difference 1 (D1)"] ("Sensor Term")
                n41 = Unbundle By Name(w177) -> ("sum1Term"=w175:T9)
                n42 = call <vilib>:"CTRE_Phoenix_MotorControl_ConfigSensorTerm_Enhanced.vi"("timeoutMs"=w173, "Sensor Term"=w174, "Feedback Device"=w175, "PhoenixMotorControlDevRef"=w176) -> ("error out"=w171:errorcluster, "PhoenixMotorControlDevRef"=w172:T12)  [unwired: 6 in]
              }
            }
          }
          frame 10 {
            # "Config Diff 0"
            n43 = Unbundle By Name(w179) -> ("diff0Term"=w178:bool)
            n44 = case shown="True" w178 {
              tunnel: w184 -> [w186 w191]
              tunnel: [w186 w190] -> w183
              tunnel: w182 -> [_ w189]
              tunnel: [errorcluster {"status"=FALSE, "code"=0, "source"=""} ("error out") w188] -> w181
              tunnel: w180 -> [_ w187]
              frame False {
              }
              frame True {
                w192 = u16 2 items=["Sum 0 (S0)", "Sum 1 (S1)", "Difference 0 (D0)", "Difference 1 (D1)"] ("Sensor Term")
                n45 = Unbundle By Name(w187) -> ("diff0Term"=w193:T9)
                n46 = call <vilib>:"CTRE_Phoenix_MotorControl_ConfigSensorTerm_Enhanced.vi"("timeoutMs"=w189, "Sensor Term"=w192, "Feedback Device"=w193, "PhoenixMotorControlDevRef"=w191) -> ("error out"=w188:errorcluster, "PhoenixMotorControlDevRef"=w190:T12)  [unwired: 6 in]
              }
            }
          }
          frame 11 {
            # "Config Diff 1"
            n47 = Unbundle By Name(w195) -> ("diff1Term"=w194:bool)
            n48 = case shown="True" w194 {
              tunnel: w200 -> [w202 w207]
              tunnel: w199 -> [_ w206]
              tunnel: w198 -> [_ w205]
              tunnel: [w202 w204] -> w197
              tunnel: [errorcluster {"status"=FALSE, "code"=0, "source"=""} ("error out") w203] -> w196
              frame False {
              }
              frame True {
                w208 = u16 3 items=["Sum 0 (S0)", "Sum 1 (S1)", "Difference 0 (D0)", "Difference 1 (D1)"] ("Sensor Term")
                n49 = Unbundle By Name(w206) -> ("diff1Term"=w209:T9)
                n50 = call <vilib>:"CTRE_Phoenix_MotorControl_ConfigSensorTerm_Enhanced.vi"("timeoutMs"=w205, "Sensor Term"=w208, "Feedback Device"=w209, "PhoenixMotorControlDevRef"=w207) -> ("error out"=w203:errorcluster, "PhoenixMotorControlDevRef"=w204:T12)  [unwired: 6 in]
              }
            }
          }
          frame 12 {
            # "Config Peak Current"
            n51 = Unbundle By Name(w213) -> ("peakCurrentLimit"=w211:bool, "peakCurrentDuration"=w212:bool)
            n52 = Or(x=w211, y=w212) -> (x .or. y?=w210:bool)
            n53 = case shown="True" w210 {
              tunnel: w218 -> [w220 w227]
              tunnel: [w220 w226] -> w217
              tunnel: w216 -> [_ w225]
              tunnel: w215 -> [_ w222]
              tunnel: [errorcluster {"status"=FALSE, "code"=0, "source"=""} ("error out") w221] -> w214
              frame False {
              }
              frame True {
                n54 = Unbundle By Name(w225) -> ("peakCurrentLimit"=w224:i32, "peakCurrentDuration"=w223:i32)
                n55 = call <vilib>:"CTRE_Phoenix_MotorControl_ConfigPeakCurrentLimit.vi"("timeoutMs"=w222, "Peak Current Maximum Duration (ms)"=w223, "Peak Current (Amps)"=w224, "PhoenixMotorControlDevRef"=w227) -> ("error out"=w221:errorcluster, "PhoenixMotorControlDevRef"=w226:T12)  [unwired: 6 in]
              }
            }
          }
          frame 13 {
            n56 = Unbundle By Name(w229) -> ("continuousCurrentLimit"=w228:bool)
            n57 = case shown="True" w228 {
              tunnel: w234 -> [_ w242]
              tunnel: w233 -> [w236 w241]
              tunnel: [w236 w239] -> w232
              tunnel: [errorcluster {"status"=FALSE, "code"=0, "source"=""} ("error out") w238] -> w231
              tunnel: w230 -> [_ w237]
              frame False {
              }
              frame True {
                n58 = Unbundle By Name(w242) -> ("continuousCurrentLimit"=w240:i32)
                n59 = call <vilib>:"CTRE_Phoenix_MotorControl_ConfigContinuousCurrentLimit.vi"("timeoutMs"=w237, "Continuous Current Limit (Amps)"=w240, "PhoenixMotorControlDevRef"=w241) -> ("error out"=w238:errorcluster, "PhoenixMotorControlDevRef"=w239:T12)  [unwired: 7 in]
              }
            }
          }
          frame Default {
          }
        }
      }
      n60 = Or Array Elements(Boolean array=w16) -> (logical OR=w15:bool)
      n61 = Select(t=errorcluster {"status"=TRUE, "code"=-1, "source"="Motor Controller Configure All Settings Enhanced: 1 or more configs failed"} ("error out 2"), s=w15, f=errorcluster {"status"=FALSE, "code"=0, "source"=""} ("error out 2")) -> (s? t:f=w22:errorcluster)
    }
    frame Error {
    }
  }
  "PhoenixMotorControlDevRef" <- w6
  "error out" <- w10
